vi "Initialize Symbols.vi"(8 "error in (no error)":errorcluster, 11 "MCLBSelection in":refnum<class "MulticolumnListboxSelection.lvclass">) -> (0 "error out":errorcluster, 3 "MCLBSelection out":refnum<class "MulticolumnListboxSelection.lvclass">)   [LabVIEW 2015, in "MulticolumnListboxSelection.lvclass"]
doc: "<b> </b> <b> </b>\n©2016 Q Software Innovations, LLC (QSI)\nwritten by Quentin Alldredge\nproduced in LabVIEW 2015\n\nsupport@qsoftwareinnovations.com\nwww.qsoftwareinnovations.com\n\nAll rights reserved.\n\nRedistribution and use in source and binary forms, with or without modification, are permitted provided that the following conditions are met:\n\n * Redistributions of source code must retain the above copyright notice, this list of conditions and the following disclaimer.\n * Redistributions in binary form must reproduce the above copyright notice, this list of conditions and the following disclaimer in the documentation and/or other materials provided with the distribution.\n * Neither the name of Q Software Innovations, LLC. nor the names of its contributors may be used to endorse or promote products derived from this software without specific prior written permission.\n\nTHIS SOFTWARE IS PROVIDED BY THE COPYRIGHT HOLDERS AND CONTRIBUTORS \"AS IS\" AND ANY EXPRESS OR IMPLIED WARRANTIES, INCLUDING, BUT NOT LIMITED TO, THE IMPLIED WARRANTIES OF MERCHANTABILITY AND FITNESS FOR A PARTICULAR PURPOSE ARE DISCLAIMED. IN NO EVENT SHALL THE COPYRIGHT OWNER OR CONTRIBUTORS BE LIABLE FOR ANY DIRECT, INDIRECT, INCIDENTAL, SPECIAL, EXEMPLARY, OR CONSEQUENTIAL DAMAGES (INCLUDING, BUT NOT LIMITED TO, PROCUREMENT OF SUBSTITUTE GOODS OR SERVICES; LOSS OF USE, DATA, OR PROFITS; OR BUSINESS INTERRUPTION) HOWEVER CAUSED AND ON ANY THEORY OF LIABILITY, WHETHER IN CONTRACT, STRICT LIABILITY, OR TORT (INCLUDING NEGLIGENCE OR OTHERWISE) ARISING IN ANY WAY OUT OF THE USE OF THIS SOFTWARE, EVEN IF ADVISED OF THE POSSIBILITY OF SUCH DAMAGE."
uses:
  MulticolumnListboxSelection.lvclass
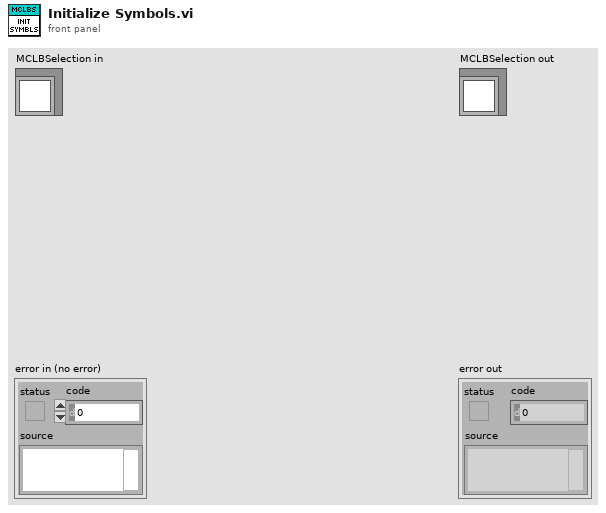
[diagram p1: front panel]
types:
  T1 = typedef "imagedata.ctl" = cluster{"image type":i32, "image depth":i32, "image":u8[], "mask":u8[], "colors":u32[], "Rectangle":cluster{"left":i16, "top":i16, "right":i16, "bottom":i16}}
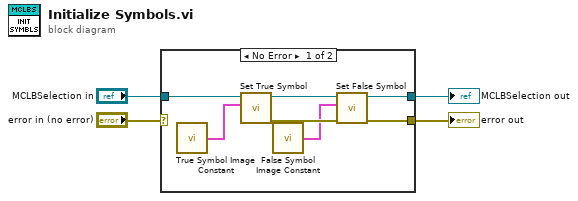
[diagram p0: block diagram]
diagram:
  n1 = case shown="No Error" "error in (no error)" {
    selector: "error in (no error)" -> [_ w13]
    tunnel: [w5 w13] -> w3
    tunnel: [w9 w12] -> w1
    tunnel: "MCLBSelection in" -> [w10 w12]
    frame No Error {
      n2 = call "True Symbol Image Constant.vi"() -> ("True Symbol Image Contant"=w7:T1)  [unwired: 5 in]
      n3 = call "Set True Symbol.vi"("True Symbol Image"=w7, "MCLBSelection in"=w10) -> ("error out"=w8:errorcluster, "MCLBSelection out"=w11:refnum<class "MulticolumnListboxSelection.lvclass">)  [unwired: 8 in]
      n4 = call "False Symbol Image Constant.vi"() -> ("False Symbol Image Constant"=w6:T1)  [unwired: 5 in]
      n5 = call "Set False Symbol.vi"("error in (no error)"=w8, "False Symbol Image"=w6, "MCLBSelection in"=w11) -> ("error out"=w5:errorcluster, "MCLBSelection out"=w9:refnum<class "MulticolumnListboxSelection.lvclass">)  [unwired: 7 in]
    }
    frame Error {
    }
  }
  "error out" <- w3
  "MCLBSelection out" <- w1
